vi "_Connect_DB.vi"(8 "error in (no error)":errorcluster, 11 "Postgres Connector In":refnum<class "Postgres Connector.lvclass">) -> (0 "error out":errorcluster, 3 "Postgres Connector Out":refnum<class "Postgres Connector.lvclass">)   [LabVIEW 2020, in "Postgres Connector.lvclass"]
doc: "This VI build the string so the user can connect to the database."
uses:
  Postgres Connector.lvclass
  Postgres Connector.lvclass/Postgres Connector.ctl
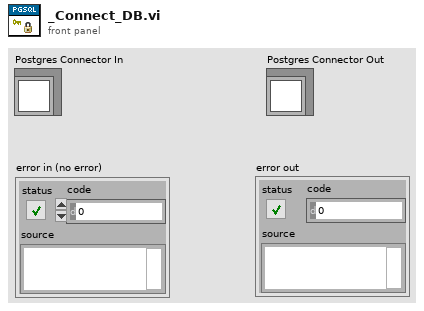
[diagram p1: front panel]
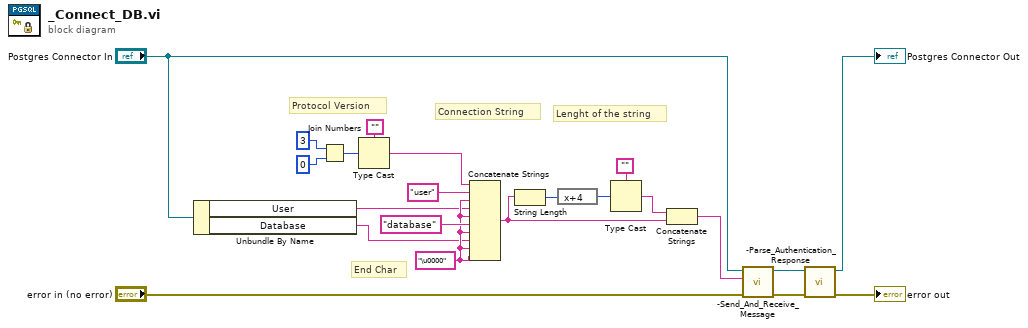
[diagram p0: block diagram]
diagram:
  w8 = "\u0000"
  # "Lenght of the string"
  # "Connection String"
  # "Protocol Version"
  # "End Char"
  n1 = Unbundle By Name("Postgres Connector In") -> ("User"=w7:string, "Database"=w6:string)
  n2 = Join Numbers(hi=i16 3, lo=i16 0) -> ((hi.lo)=w14:u32)
  n3 = Type Cast(type="", x=w14) -> (*(type *) &x=w12:string)
  n4 = Concatenate Strings(w12, "user", w8, w7, w8, "database", w8, w6, w8, w8) -> (w9:string)
  n5 = String Length(string=w9) -> (length=w2:i32)
  n6 = expression code="x+4"(w2) -> (w1:i32)
  n7 = Type Cast(type="", x=w1) -> (*(type *) &x=w10:string)
  n8 = Concatenate Strings(w10, w9) -> (w5:string)
  n9 = call "-Send_And_Receive_Message.vi"("error in (no error)"="error in (no error)", "Message To Send"=w5, "Postgres Connector In"="Postgres Connector In") -> ("error out"=w4:errorcluster, "Postgres Connector Out"=w3:refnum<class "Postgres Connector.lvclass">)  [unwired: 7 in]
  n10 = call "-Parse_Authentication_Response.vi"("error in (no error)"=w4, "Postgres Connector In"=w3) -> ("error out"=→"error out":errorcluster, "Postgres Connector Out"=→"Postgres Connector Out":refnum<class "Postgres Connector.lvclass">)  [unwired: 8 in]
